vi "Suck ball.vi"(0 "Intake Info In":T2, 1 "Kick Info":T1, 2 "error in (no error)":errorcluster) -> (3 "Intake Info Out":T2, 4 "Kick Info":T1, 5 "Finished?":bool, 6 "error out":errorcluster)   [LabVIEW 2013]
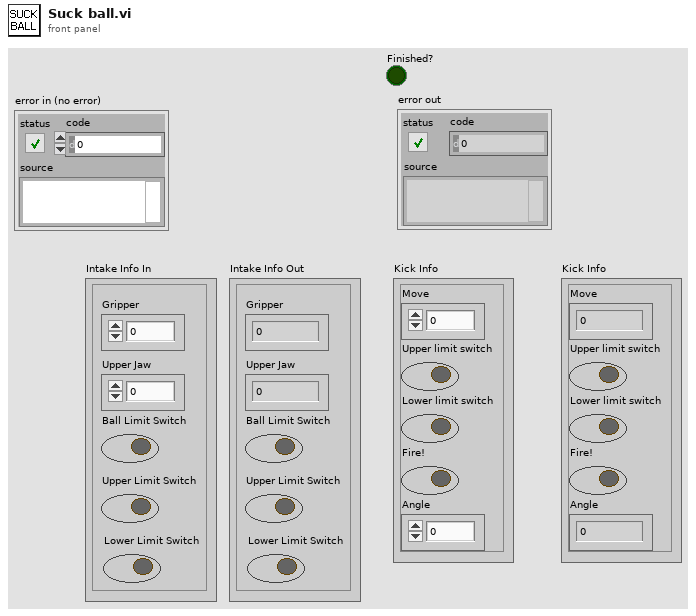
[diagram p1: front panel]
types:
  T1 = cluster{"Move":dbl, "Upper limit switch":bool, "Lower limit switch ":bool, "Fire!":bool, "Angle":dbl}
  T2 = cluster{"Gripper":dbl, "Upper Jaw":dbl, "Ball Limit Switch":bool, "Upper Limit Switch":bool, "Lower Limit Switch ":bool}
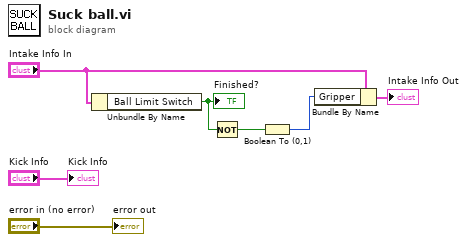
[diagram p0: block diagram]
diagram:
  n1 = Unbundle By Name("Intake Info In") -> ("Ball Limit Switch"=w1:bool)
  "Finished?" <- w1
  n2 = Not(x=w1) -> (.not. x?=w6:bool)
  n3 = Boolean To (0,1)(Boolean=w6) -> (0, 1=w5:i16)
  n4 = Bundle By Name(cluster="Intake Info In", "Gripper"=w5) -> (→"Intake Info Out":T2)
  "error out" <- "error in (no error)"
  "Kick Info" <- "Kick Info"
